vi "Initiate Pulse Test.vi"(7 "Pulse Number (0: Single Pulse)":i32(ring) items=["Single Pulse", "Dual Pulse"], 8 "error in (no error)":errorcluster, 9 "Pulse Train Tag 2 (2)":i32=2, 10 "Pulse Train Tag 1 (1)":i32=1, 11 "VISA resource name":refnum<visa-resource-name>) -> (0 "error out":errorcluster, 3 "VISA resource name out":refnum<visa-resource-name>)   [LabVIEW 2015, in "Keithley 2600 Series.lvlib"]
doc: "Initiates the pulse configuration assigned to pulse train tag.\n\n<b>Notes:</b>\n(1) Configures the pulse train by <b>Configure Tag Current Pulse </b>VI or <b>Configure Tag Voltage Pulse </b>VI before initiating it.\n(2) Turns off the autozero mode by <b>Configure Measurement Characteristics </b>VI before you call This VI.\n(3) Turns off the measure auto range mode by <b>Configure Measurement Range </b>VI before you call This VI.\n(4) Turns off the source auto range mode by <b>Configure Source (Range) </b>VI before you call This VI.\n(5) If initiate dual pulse the pulse train of tag 1 and tag 2 must use different channel and each channel must use a separate buffer of measurement."
uses:
  Keithley 2600 Series.lvlib
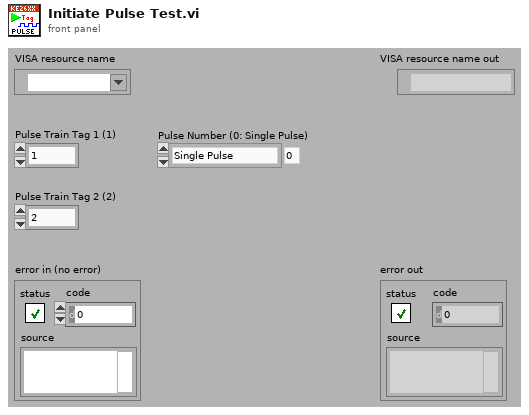
[diagram p1: front panel]
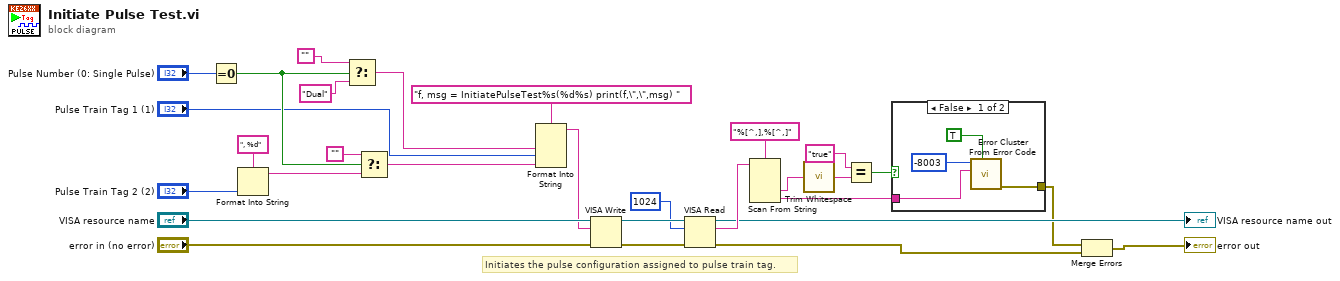
[diagram p0: block diagram]
diagram:
  # "Initiates the pulse configuration assigned to pulse train tag."
  n1 = Equal To 0?(x="Pulse Number (0: Single Pulse)") -> (x = 0?=w7:bool)
  n2 = Format Into String(format string=", %d", "Pulse Train Tag 2 (2)") -> (resulting string=w22:string)  [unwired: 2 in, 1 out]
  n3 = Select(t="", s=w7, f="Dual") -> (s? t:f=w4:string)
  n4 = Select(t="", s=w7, f=w22) -> (s? t:f=w3:string)
  n5 = Format Into String(format string="f, msg = InitiatePulseTest%s(%d%s) print(f,\",\",msg) ", w4, "Pulse Train Tag 1 (1)", w3) -> (resulting string=w21:string)  [unwired: 2 in, 1 out]
  n6 = VISA Write(VISA resource name="VISA resource name", write buffer=w21, error in (no error)="error in (no error)") -> (VISA resource name out=w20:refnum<visa-resource-name>, error out=w19:errorcluster)  [unwired: 1 out]
  n7 = VISA Read(VISA resource name=w20, byte count=u32 1024, error in (no error)=w19) -> (VISA resource name out=→"VISA resource name out":refnum<visa-resource-name>, read buffer=w17:string, error out=w2:errorcluster)  [unwired: 1 out]
  n8 = Scan From String(format string="%[^,],%[^,]", input string=w17) -> (output 1=w11:string, output 2=w13:string)  [unwired: 4 in, 3 out]
  n9 = call <vilib>:"Trim Whitespace.vi"("string"=w11) -> ("trimmed string"=w12:string)  [unwired: 1 in]
  n10 = Equal?(x="true", y=w12) -> (x = y?=w14:bool)
  n11 = case shown="False" w14 {
    tunnel: [w32 _] -> w1
    tunnel: w13 -> [w31 _]
    frame False {
      n12 = call <vilib>:"Error Cluster From Error Code.vi"("show call chain? (False)"=TRUE, "error message (\"\")"=w31, "error code (0)"=-8003) -> ("error out"=w32:errorcluster)  [unwired: 6 in]
    }
    frame True {
    }
  }
  n13 = Merge Errors(w1, w2) -> (→"error out":errorcluster)
